vi "ReceiveTCPfromPi.vi"() -> ()   [LabVIEW 2014]
panel:
  out "output cluster":T1
  in  "Datalog File":path=path "C:/Users/romneyj/Desktop/EKFDatalog.txt"
  out "length 2":i32
  out "length":i32
  in  "Values to Display 2":dbl(slide)=100.0 min=10.0 max=2000.0 step=10.0 scale=10.0..2000.0
  out "error out":errorcluster
  out "before substring":string
  out "Roll":cluster{dbl, dbl}(graph)
  out "Pitch":cluster{dbl, dbl}(graph)
  out "Yaw":cluster{dbl, dbl}(graph)
  in  "stop":bool
  in  "Port":u16=5005
  in  "IP Address":string="155.31.242.65"
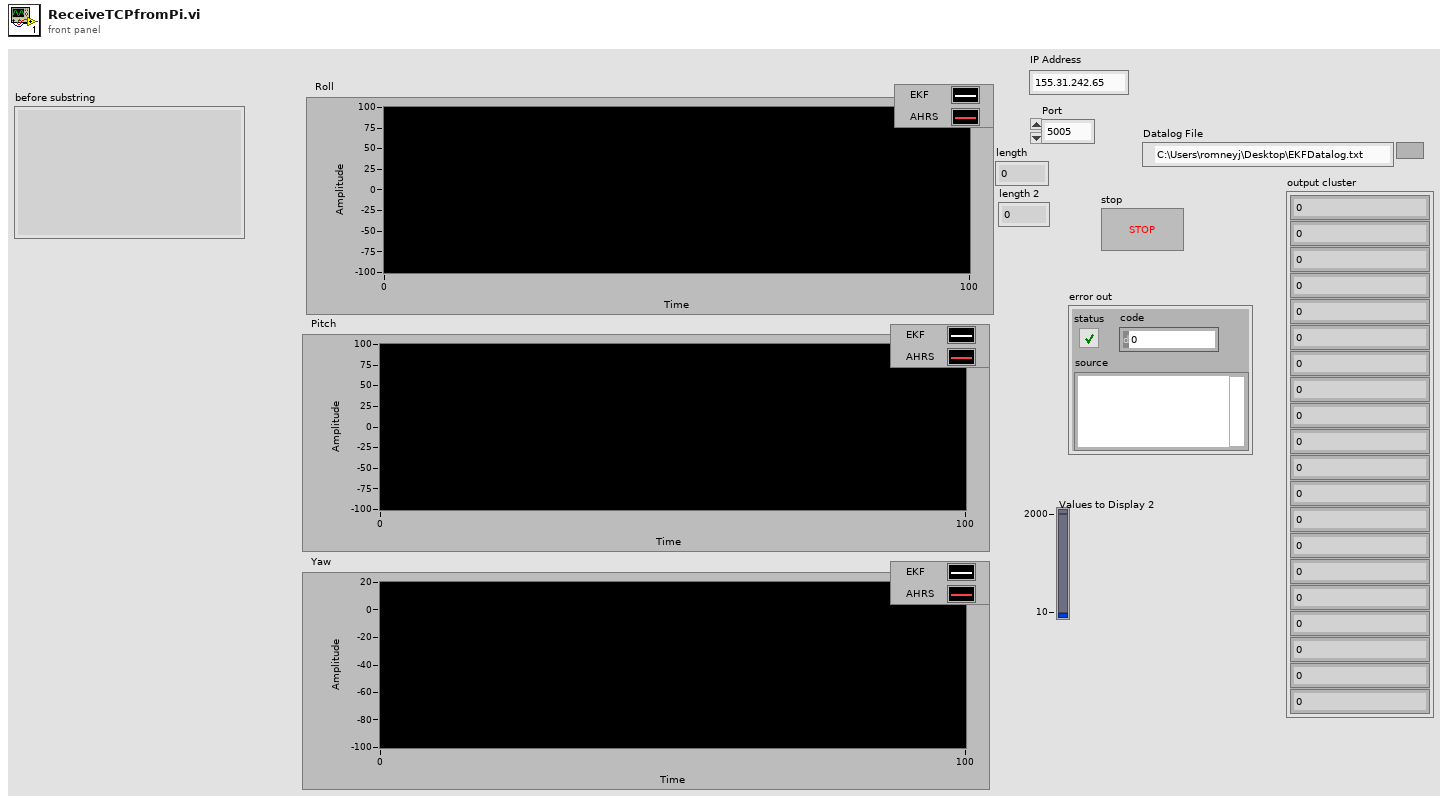
[diagram p1: front panel]
types:
  T1 = cluster{dbl, dbl, dbl, dbl, dbl, dbl, dbl, dbl, dbl, dbl, i32, dbl, dbl, dbl, dbl, dbl, dbl, dbl, dbl, dbl}
  T2 = enum16{"open", "replace", "create", "open or create", "replace or create", "replace or create with confirmation"}
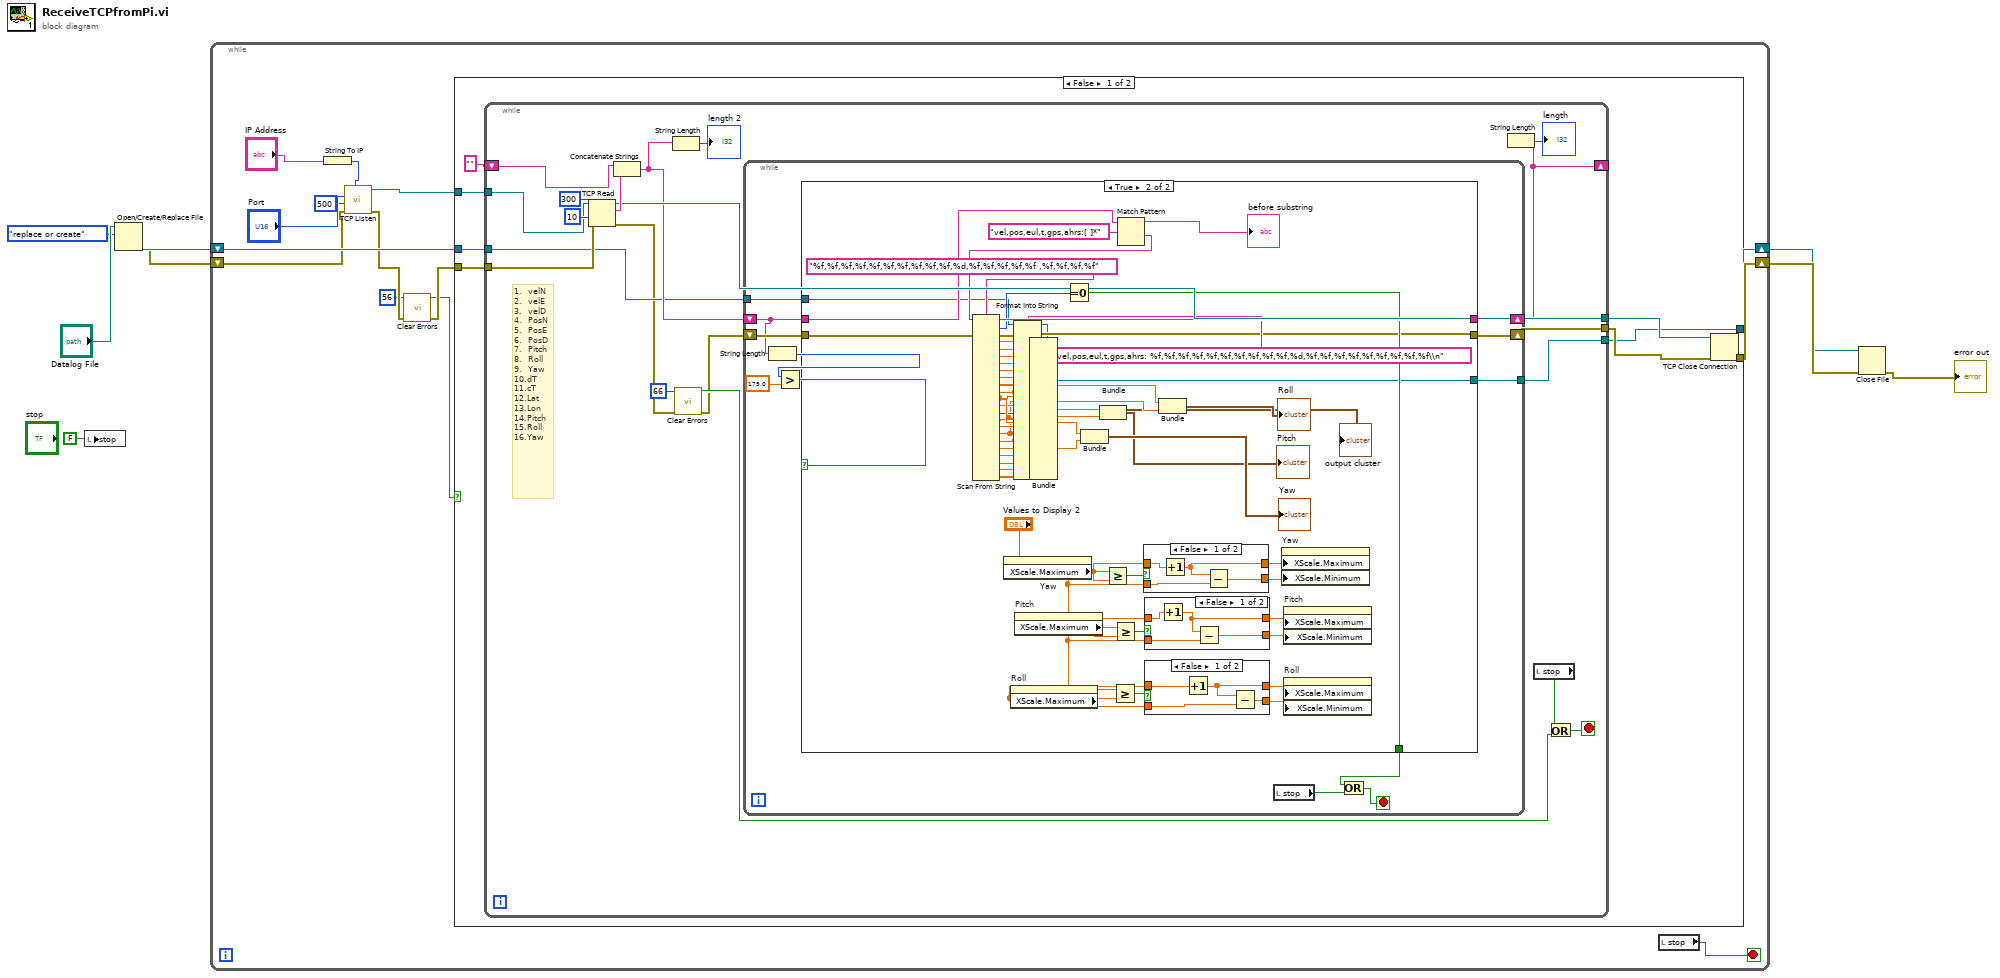
[diagram p0: block diagram]
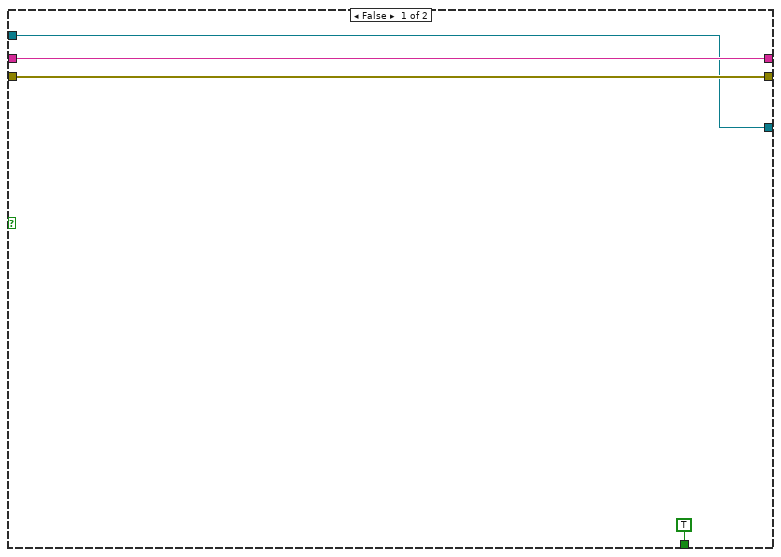
[diagram p2: hidden frame]
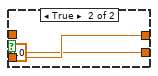
[diagram p3: hidden frame]
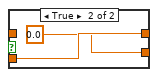
[diagram p4: hidden frame]
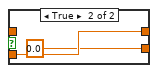
[diagram p5: hidden frame]
diagram:
  n1 = local write "stop"(FALSE ("stop")) -> ()
  n2 = Open/Create/Replace File(file path (use dialog)="Datalog File", operation (0:open)=T2."replace or create") -> (refnum out=w6:refnum<file>, error out=w4:errorcluster)  [unwired: 4 in, 1 out]
  n3 = while {
    shift-right: [w15] -> w1
    shift-left: w6 -> [w18]
    shift-right: [w16] -> w3
    shift-left: w4 -> [w17]
    stop <- w14 stop-if-true
    n4 = String To IP(1:"IP Address") -> (0:w20:u32)
    n5 = call <vilib>:"TCP Listen.vi"("net address"=w20, "error in (no error)"=w17, "timeout ms (wait forever: -1)"=500, "port"="Port") -> ("error out"=w12:errorcluster, "connection ID"=w19:refnum<k5>)  [unwired: 3 in, 3 out]
    n6 = call <vilib>:"Clear Errors.vi"("error in (no error)"=w12, "specific error code to clear (0: all)"=56) -> ("error out"=w11:errorcluster, "specific error cleared?"=w9:bool)  [unwired: 4 in]
    n7 = case shown="False" w9 {
      tunnel: w19 -> [w30 _]
      tunnel: w18 -> [w27 w136]
      tunnel: [w25 w137] -> w16
      tunnel: [w24 w136] -> w15
      tunnel: w11 -> [w23 w137]
      frame False {
        n8 = while {
          tunnel: w30 -> [w47]
          tunnel: w23 -> [w46]
          shift-right: [w40] -> _
          shift-left: "" -> [w45]
          tunnel: [w44] -> w28
          tunnel: [w43] -> w26
          tunnel: w27 -> [w38]
          tunnel: [w37] -> w24
          stop <- w33 stop-if-true
          # "1.  velN\n2.  velE\n3.  velD\n4.  PosN\n5.  PosE\n6.  PosD\n7.  Pitch\n8.  Roll\n9.  Yaw\n10.dT\n11.cT\n12.Lat\n13.Lon\n14.Pitch\n15.Roll\n16.Yaw"
          n9 = TCP Read(connection ID=w47, bytes to read=300, error in (no error)=w46, 9:10 ("timeout ms (25000)")) -> (connection ID out=w44:refnum<k5>, data out=w50:string, error out=w32:errorcluster)  [unwired: 1 in]
          n10 = Concatenate Strings(w45, w50) -> (w39:string)
          n11 = String Length(string=w39) -> (length=→"length 2":i32)
          n12 = call <vilib>:"Clear Errors.vi"("error in (no error)"=w32, "specific error code to clear (0: all)"=66 ("error code (no error:0)")) -> ("error out"=w31:errorcluster, "specific error cleared?"=w34:bool)  [unwired: 4 in]
          n13 = while {
            shift-right: [w61] -> w43
            shift-left: w31 -> [w62]
            shift-right: [w60] -> w40
            shift-left: w39 -> [w55]
            tunnel: w38 -> [w52]
            tunnel: [w51] -> w37
            stop <- w57 stop-if-true
            n14 = String Length(string=w55) -> (length=w54:i32)
            n15 = Greater?(x=w54, y=175.0) -> (0:w53:bool)
            n16 = case shown="True" w53 {
              tunnel: w62 -> [w64 w116]
              tunnel: w55 -> [w65 w114]
              tunnel: [w64 w89] -> w61
              tunnel: [w65 w96] -> w60
              tunnel: [TRUE w94] -> w59
              tunnel: w52 -> [w63 w90]
              tunnel: [w63 w88] -> w51
              frame False {
              }
              frame True {
                n17 = property on="Yaw" class="WFChart (strict)"() -> ("XScale.Maximum"=w108:dbl)  [unwired: 2 in, 2 out]
                n18 = property on="Roll" class="WFChart (strict)"() -> ("XScale.Maximum"=w100:dbl)  [unwired: 2 in, 2 out]
                n19 = property on="Pitch" class="WFChart (strict)"() -> ("XScale.Maximum"=w103:dbl)  [unwired: 2 in, 2 out]
                n20 = Greater Or Equal?(x="Values to Display 2", y=w108) -> (x >= y?=w109:bool)
                n21 = Greater Or Equal?(x="Values to Display 2", y=w100) -> (x >= y?=w104:bool)
                n22 = Greater Or Equal?(x="Values to Display 2", y=w103) -> (x >= y?=w105:bool)
                n23 = Match Pattern(string=w114, regular expression="vel,pos,eul,t,gps,ahrs:[ ]*") -> (before substring=→"before substring":string, after substring=w115:string)  [unwired: 1 in, 2 out]
                n24 = Scan From String(format string="%f,%f,%f,%f,%f,%f,%f,%f,%f,%f,%d,%f,%f,%f,%f,%f ,%f,%f,%f,%f", input string=w115, error in=w116) -> (remaining string=w96:string, offset past scan=w95:u32, error out=w91:errorcluster, output 1=w87:dbl, output 2=w86:dbl, output 3=w85:dbl, output 4=w84:dbl, output 5=w83:dbl, output 6=w82:dbl, output 7=w81:dbl, output 8=w80:dbl, output 9=w79:dbl, output 10=w78:dbl, output 11=w77:i32, output 12=w76:dbl, output 13=w75:dbl, output 14=w74:dbl, output 15=w73:dbl, output 16=w72:dbl, output 17=w71:dbl, output 18=w70:dbl, output 19=w69:dbl, output 20=w68:dbl)  [unwired: 21 in]
                n25 = Format Into String(format string="vel,pos,eul,t,gps,ahrs: %f,%f,%f,%f,%f,%f,%f,%f,%f,%f,%d,%f,%f,%f,%f,%f,%f,%f,%f,%f\\n", initial string=w90, error in=w91, w87, w86, w85, w84, w83, w82, w81, w80, w79, w78, w77, w76, w75, w74, w73, w72, w71, w70, w69, w68) -> (resulting string=w88:refnum<file>, error out=w89:errorcluster)
                n26 = Bundle(w87, w86, w85, w84, w83, w82, w81, w80, w79, w78, w77, w76, w75, w74, w73, w72, w71, w70, w69, w68) -> (→"output cluster":T1)  [unwired: 1 in]
                n27 = Equal To 0?(x=w95) -> (x = 0?=w94:bool)
                n28 = Bundle(w79, w72) -> (→"Yaw":cluster{dbl, dbl})  [unwired: 1 in]
                n29 = Bundle(w80, w73) -> (→"Pitch":cluster{dbl, dbl})  [unwired: 1 in]
                n30 = case shown="False" w109 {
                  tunnel: "Values to Display 2" -> [w131 w135]
                  tunnel: w108 -> [w133 _]
                  tunnel: [w130 w135] -> w107
                  tunnel: [w132 0.0] -> w106
                  frame False {
                    n31 = Increment(x=w133) -> (x+1=w130:dbl)
                    n32 = Subtract(x=w130, y=w131) -> (x-y=w132:dbl)
                  }
                  frame True {
                  }
                }
                n33 = case shown="False" w105 {
                  tunnel: "Values to Display 2" -> [w125 w129]
                  tunnel: w103 -> [w127 _]
                  tunnel: [w124 w129] -> w102
                  tunnel: [w126 0.0] -> w101
                  frame False {
                    n34 = Increment(x=w127) -> (x+1=w124:dbl)
                    n35 = Subtract(x=w124, y=w125) -> (x-y=w126:dbl)
                  }
                  frame True {
                  }
                }
                n36 = case shown="False" w104 {
                  tunnel: "Values to Display 2" -> [w119 w123]
                  tunnel: w100 -> [w121 _]
                  tunnel: [w118 w123] -> w99
                  tunnel: [w120 0.0] -> w98
                  frame False {
                    n37 = Increment(x=w121) -> (x+1=w118:dbl)
                    n38 = Subtract(x=w118, y=w119) -> (x-y=w120:dbl)
                  }
                  frame True {
                  }
                }
                n39 = Bundle(w81, w74) -> (→"Roll":cluster{dbl, dbl})  [unwired: 1 in]
                n40 = property on="Yaw" class="WFChart (strict)"("XScale.Maximum"=w107, "XScale.Minimum"=w106) -> ()  [unwired: 2 in, 2 out]
                n41 = property on="Pitch" class="WFChart (strict)"("XScale.Maximum"=w102, "XScale.Minimum"=w101) -> ()  [unwired: 2 in, 2 out]
                n42 = property on="Roll" class="WFChart (strict)"("XScale.Maximum"=w99, "XScale.Minimum"=w98) -> ()  [unwired: 2 in, 2 out]
              }
            }
            n43 = local read "stop"() -> (w58:bool)
            n44 = Or(x=w59, y=w58) -> (x .or. y?=w57:bool)
          }
          n45 = String Length(string=w40) -> (length=→"length":i32)
          n46 = local read "stop"() -> (w35:bool)
          n47 = Or(x=w35, y=w34) -> (x .or. y?=w33:bool)
        }
        n48 = TCP Close Connection(connection ID=w28, error in (no error)=w26) -> (error out=w25:errorcluster)  [unwired: 1 in, 1 out]
      }
      frame True {
      }
    }
    n49 = local read "stop"() -> (w14:bool)
  }
  n50 = Close File(refnum=w1, error in=w3) -> (error out=→"error out":errorcluster)  [unwired: 1 out]
